vi "Test.Mathematica.vi"() -> ()   [LabVIEW 2014]
uses:
  D:/GitHub/iontrapnet/Mathematica/Wolfram.NETLink.dll
  Wolfram.NETLink.dll
panel:
  out "Mathematica":refnum<k24>
  in  "Script":path=path "Test.m"
  in  "Test":bool caption="stop"
  in  "Content":string
  in  "Path":path
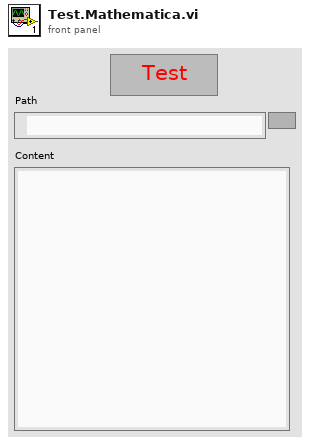
[diagram p1: front panel]
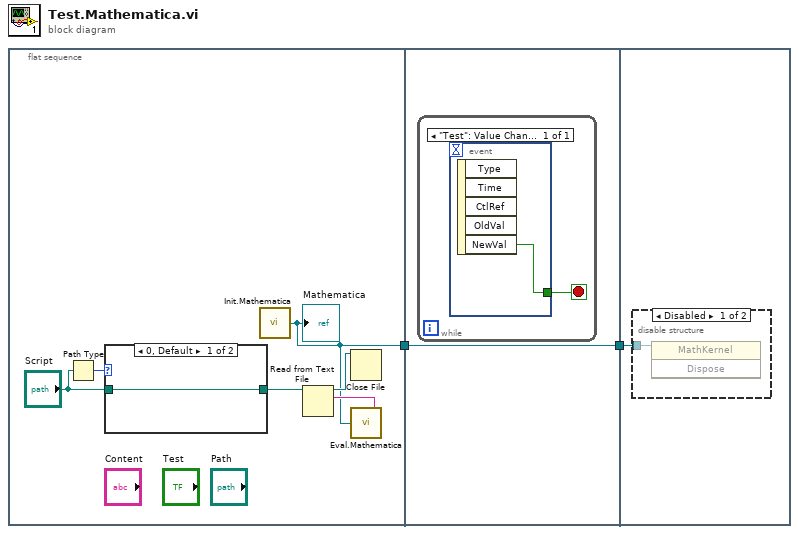
[diagram p0: block diagram]
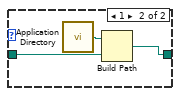
[diagram p2: hidden frame]
diagram:
  n1 = flat-sequence {
    tunnel: [w6] -> w1
    tunnel: [w13] -> w2
    tunnel: w1 -> [w13]
    tunnel: w2 -> [w16]
    frame #0 {
      n2 = Path Type(1:"Script") -> (0:w5:i16)
      n3 = case shown="0, Default" w5 {
        tunnel: "Script" -> [w9 w10]
        tunnel: [w9 w11] -> w3
        frame 0, Default {
        }
        frame 1 {
          n4 = call <vilib>:"Application Directory.vi"() -> ("Application Directory"=w12:path)
          n5 = Build Path(base path=w12, name or relative path=w10) -> (appended path=w11:path)
        }
      }
      n6 = call "Init.Mathematica.vi"() -> ("reference"=w6:refnum<k24>)  [unwired: 1 in]
      "Mathematica" <- w6
      n7 = Read from Text File(file (use dialog)=w3) -> (refnum out=w8:refnum<file>, text=w7:string)  [unwired: 3 in, 2 out]
      n8 = Close File(refnum=w8) -> ()  [unwired: 1 in, 2 out]
      n9 = call "Eval.Mathematica.vi"("input"=w7, "reference"=w6) -> ()
    }
    frame #1 {
      n10 = while {
        stop <- w14 stop-if-true
        n11 = event shown="[0] \"Test\": Value Change" {
          selector: _ -> [_]
          dyn-events: _ -> [_]
          timeout: _ -> [_]
          tunnel: [w15] -> w14
          event "Test": Value Change {
            n12 = event-data() -> ("NewVal"=w15:bool)  [unwired: 1 in, 4 out]
          }
        }
      }
    }
    frame #2 {
      n13 = disable-structure shown="Disabled" {
        disable-tunnel: w16 -> [w17 _]
        frame Disabled {
          n14 = invoke class="MathKernel" method="Dispose"(reference=w17) -> ()  [unwired: 2 in, 3 out]
        }
        frame Enabled {
        }
      }
    }
  }
